vi "EPTxFPGA add-on test.vi"() -> ()   [LabVIEW 2019]
uses:
  <vilib>/Powertrain Controls/Device Drivers/Engine Position Tracking/EPTx/RevA/FPGA/Controls/EPTxSupervisor.ctl
  <vilib>/Powertrain Controls/Device Drivers/Engine Position Tracking/EPTx/RevA/FPGA/Controls/EPTxTooth.ctl
  <vilib>/Powertrain Controls/Device Drivers/Engine Position Tracking/EPTx/RevA/FPGA/Controls/EPTxConfig.ctl
  <vilib>/Platform/TimedLoop/XDataNode/timing_clust.ctl
  <vilib>/Platform/TimedLoop/XDataNode/nitl_modes.ctl
  <vilib>/Platform/TimedLoop/XDataNode/wakeup.ctl
  <vilib>/Powertrain Controls/Device Drivers/Engine Position Tracking/EPTx/RevA/FPGA/Controls/EPTxAAPControl.ctl
  <vilib>/Powertrain Controls/Device Drivers/Engine Position Tracking/EPTx/RevA/FPGA/Controls/EPTxSignals.ctl
  <vilib>/Powertrain Controls/Device Drivers/Engine Position Tracking/EPTx/RevA/FPGA/Controls/EPTxControl.ctl
  <vilib>/rvi/Emulation/niFpgaGetClockAttributes.vi
  <vilib>/rvi/Emulation/niFpgaSctlEmulationGetInTimedLoop.vi
  <vilib>/rvi/Emulation/niFpgaEmulationReportErrorSimple.vi
  <vilib>/rvi/Emulation/niFpgaCriticalErrorInLSC.vi
  <vilib>/rvi/eio/common/nirviEmuTemplateMethod_errors.vi
  <vilib>/rvi/interface/RandomDataEmulation/niFpgaRandomDataHandleErrors.vi
  <vilib>/eio/EIONode/EIONode.xnode
  <vilib>/rvi/DataTransferAndStorage/Container/XNode/niFpgaContainer.xnode
  <vilib>/rvi/interface/RandomDataEmulation/nirviRandomDataFpgaReadWriteTemplate.vi
  <vilib>/Platform/TimedLoop/XDataNode/XDataNode.xnode
  <vilib>/Powertrain Controls/Device Drivers/Engine Position Tracking/EPTx/RevA/FPGA/EPTx - RevA - FPGA.lvlib
  <vilib>/Platform/TimedLoop/XDataNode/XDNodeRunTimeDep.lvlib
panel:
  out "AvgSpeed":fxp<+/-,64,32>
  out "CADRate":fxp<+/-,64,32>
  out "HistoryCAD":fxp<+/-,64,32>
  out "MaxCAD":fxp<+/-,64,32>
  out "CurrentCAD":fxp<+/-,64,32>
  in  "Cylinder1_H_F [CAD]":fxp<+/-,64,32>
  in  "Cylinder1_H_R [CAD]":fxp<+/-,64,32>
  in  "Sim Rate":fxp<+/-,64,32>
  in  "EPTxConfig":T1
  out "EPTxTooth":T2
  out "EPTxSupervisor":T3
  in  "Enable":bool
  in  "FallingCAD":fxp<+/-,64,32>
  in  "Cylinder1_L_R [CAD]":fxp<+,18,11> format="%.11g"
  in  "Cylinder1_L_F [CAD]":fxp<+,18,11> format="%.11g"
  out "Sync":bool
  out "Config":bool
  out "Rcvg Primary":bool
  out "Stall":bool
  out "Overflow":bool
  out "Ratio Error":bool
  out "Pattern Error":bool
  out "Aux Warning":bool
  out "Watchdog Error":bool
  in  "Sync Enable":bool
  in  "Clear Errors":bool
  in  "Sim Enable":bool
  in  "Watchdog":bool
  in  "RisingCAD":fxp<+/-,64,32>
  in  "Eng_CurSpeed":fxp<+/-,64,32>
  in  "FXP27.5":fxp<+/-,27,5>
  out "FXP27.5 out":fxp<+/-,27,5>
  in  "FXP20.5":fxp<+/-,20,5>
  out "FXP20.5 out":fxp<+/-,20,5>
  in  "FXP16.7":fxp<+/-,16,7>
  out "FXP16.7 out":fxp<+/-,16,7>
  out "FXP64.32 out":fxp<+/-,64,32>
  out "FXP32.8 out":fxp<+/-,32,8>
  out "FXP16.5 out":fxp<+/-,16,5>
  out "FXP24.5 out":fxp<+/-,24,5>
  in  "FXP64.32":fxp<+/-,64,32>
  in  "FXP32.8":fxp<+/-,32,8>
  in  "FXP16.5":fxp<+/-,16,5>
  in  "FXP24.5":fxp<+/-,24,5>
  out "Boolean 2":bool=TRUE
  out "Fast timeout":bool
  out "Med timeout":bool
  out "Slow timeout":bool
  in  "I16":i16
  in  "I8":i8
  in  "I64":i64
  in  "I32":i32
  in  "U16":u16
  in  "U8":u8
  in  "U64":u64
  in  "U32":u32
  in  "SGL":sgl
  in  "Boolean":bool
  out "I16 out":i16
  out "I8 out":i8
  out "I64 out":i64
  out "I32 out":i32
  out "U16 out":u16
  out "U8 out":u8
  out "U64 out":u64
  out "U32 out":u32
  out "SGL out":sgl
  out "Boolean out":bool
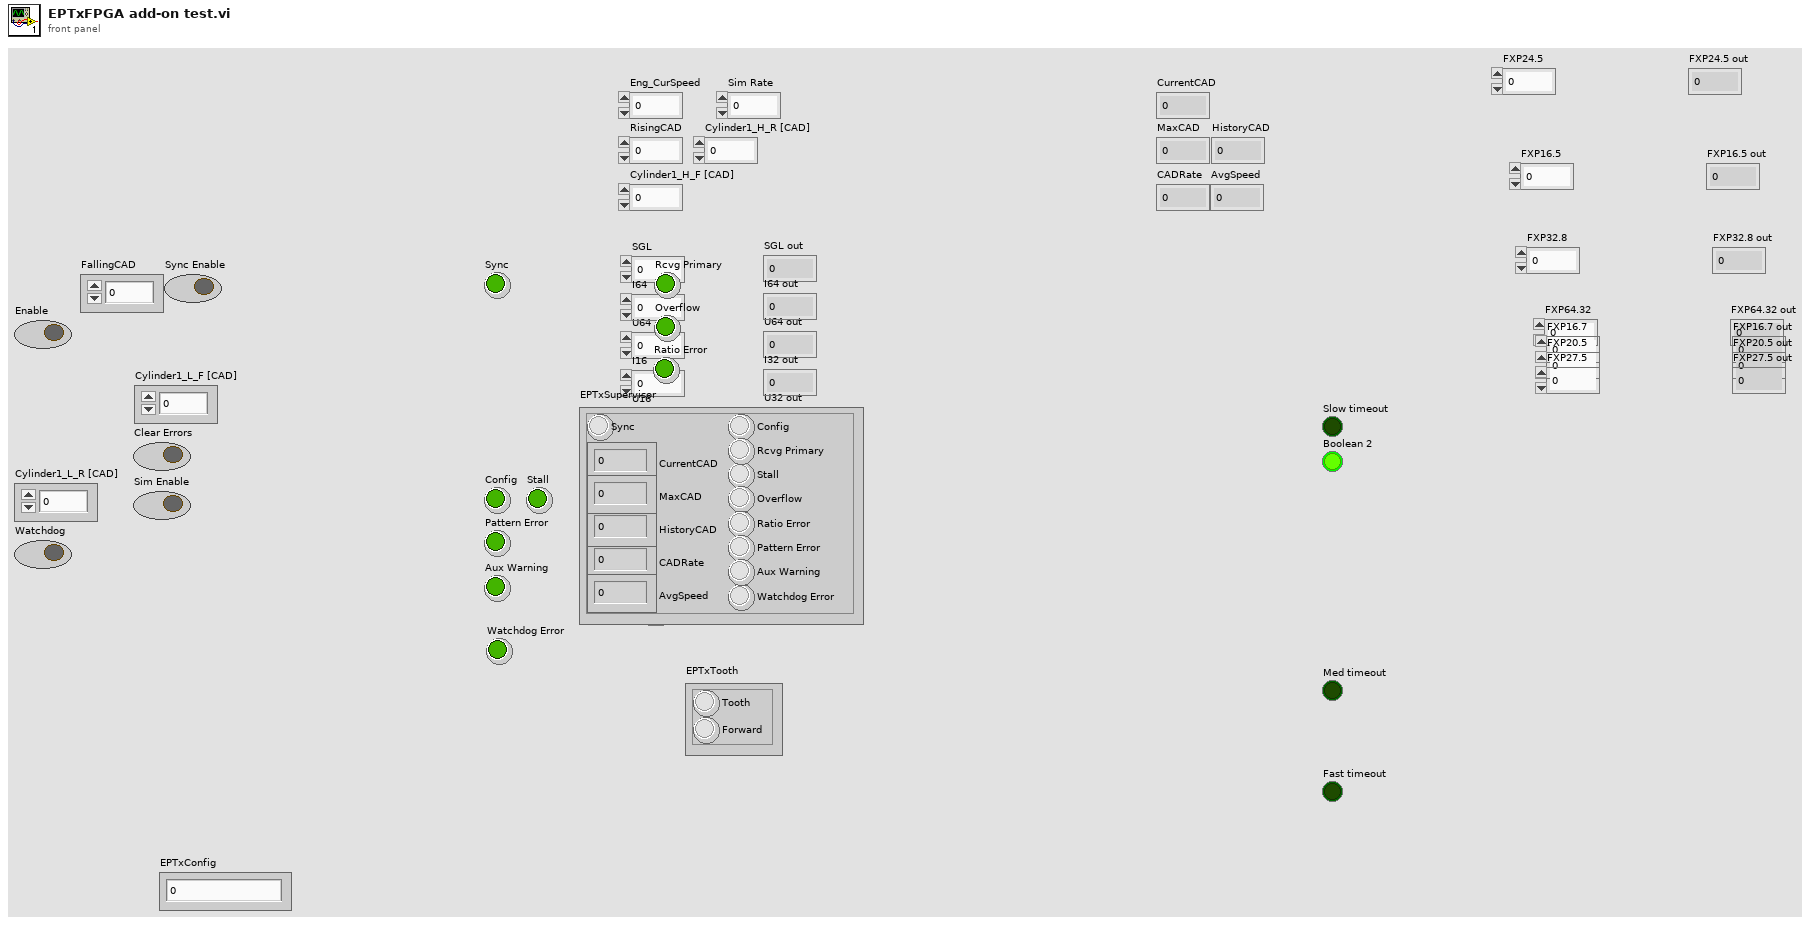
[diagram p1: front panel]
types:
  T1 = typedef "EPTx - RevA - FPGA.lvlib/EPTxConfig.ctl" = u64
  T2 = typedef "EPTx - RevA - FPGA.lvlib/EPTxTooth.ctl" = cluster{"Tooth":bool, "Forward":bool}
  T3 = typedef "EPTx - RevA - FPGA.lvlib/EPTxSupervisor.ctl" = cluster{"Sync":bool, "CurrentCAD":fxp<+,18,11>, "MaxCAD":fxp<+,11,11>, "HistoryCAD":fxp<+,11,11>, "CADRate":fxp<+,22,8>, "AvgSpeed":fxp<+,17,15>, "Config":bool, "Rcvg Primary":bool, "Stall":bool, "Overflow":bool, "Ratio Error":bool, "Pattern Error":bool, "Aux Warning":bool, "Watchdog Error":bool}
  T4 = typedef "EPTx - RevA - FPGA.lvlib/EPTxControl.ctl" = cluster{"Sync Enable":bool, "Clear Errors":bool, "Sim Enable":bool, "Sim Rate":fxp<+,24,6>, "Watchdog":bool}
  T5 = cluster{"Cylinder1_H_R [CAD]":fxp<+,18,11>, "Cylinder1_H_F [CAD]":fxp<+,18,11>, "Cylinder1_L_R [CAD]":fxp<+,18,11>, "Cylinder1_L_F [CAD]":fxp<+,18,11>}
  T6 = typedef "EPTx - RevA - FPGA.lvlib/EPTxAAPControl.ctl" = cluster{"Enable":bool, "RisingCAD":fxp<+,18,11>, "FallingCAD":fxp<+,18,11>}
  T7 = typedef "EPTx - RevA - FPGA.lvlib/EPTxSignals.ctl" = cluster{"Primary":bool, "Aux 1":bool, "Aux 2":bool, "Aux 3":bool, "Aux 4":bool}
  T8 = typedef "XDNodeRunTimeDep.lvlib/timing_clust.ctl" = cluster{"Expected End [f-1]":u64, "Actual End [f-1]":u64, "Finished Late? [f-1]":bool, "Expected End [i-1]":u64, "Actual End [i-1]":u64, "Finished Late? [i-1]":bool, "Expected Start [i]":u64, "Actual Start [i]":u64, "Expected Start [f]":u64, "Actual Start [f]":u64, "Source Name":string, "Structure Name":string, "Period":i64, "Deadline":i64, "Offset":i64, "Start":i64, "Priority":i32, "Timeout":i32, "Mode":T9, "Wakeup Reason":T10, "Error":errorcluster, "Source Type":string, "Secondary Source Type":string, "Global End Time":u64, "Global Start Time":u64, "Frame Duration":u64, "Iteration Duration":u64, "Assigned CPU":i32, "I/O Scan Engine Mode":u32}
  T9 = typedef "XDNodeRunTimeDep.lvlib/nitl_modes.ctl" = enum32{"No Change", "Process missed periods, maintain original phase", "Discard missed periods, maintain original phase", "Process missed periods, ignore original phase", "Discard missed periods, ignore original phase"}
  T10 = typedef "XDNodeRunTimeDep.lvlib/wakeup.ctl" = enum32{"Normal", "Aborted", "Asynchronous wakeup", "Timing source error", "Timed loop error", "Timeout"}
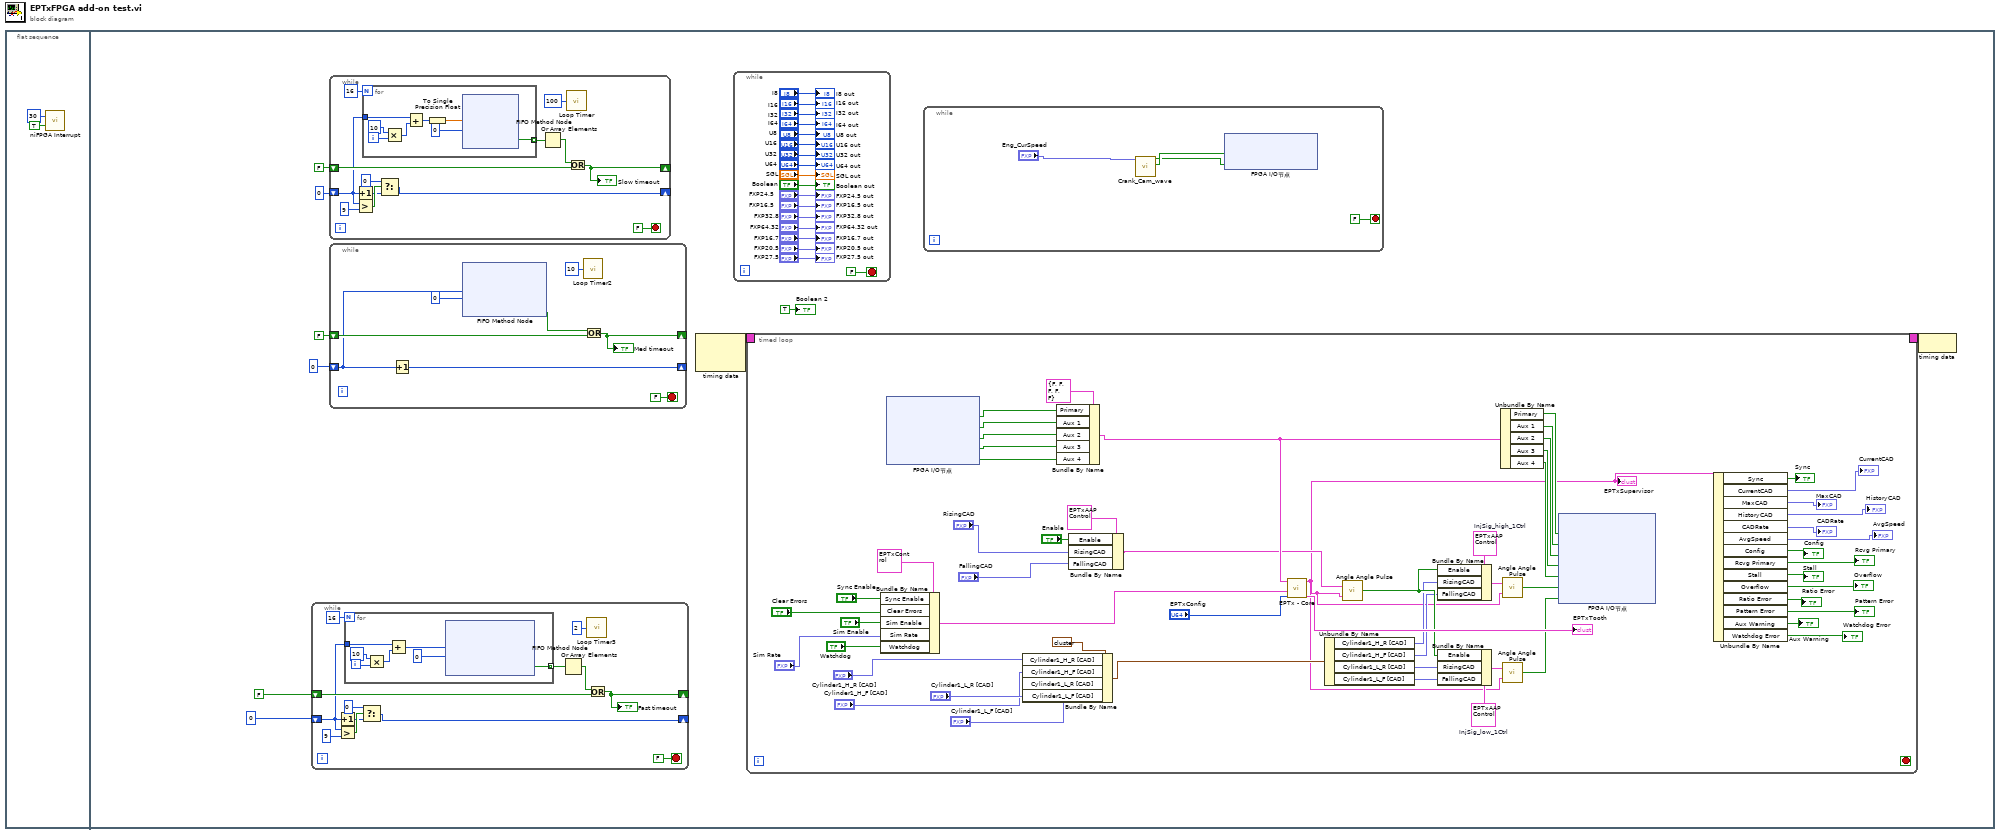
[diagram p0: block diagram]
diagram:
  n1 = flat-sequence {
    frame #0 {
      n2 = call <vilib>:"niFPGA Interrupt.vi"("Wait Until Cleared (F)"=TRUE, "IRQ Number (0)"=u8 30) -> ()  [unwired: 1 in]
    }
    frame #1 {
      n3 = while {
        shift-right: [w85] -> _
        shift-left: 0 ("t") -> [w78]
        shift-right: [w79] -> _
        shift-left: FALSE -> [w80]
        stop <- FALSE stop-if-true
        n4 = Increment(x=w78) -> (x+1=w83:i32)
        n5 = Greater?(x=w78, y=9) -> (0:w89:bool)
        n6 = for {
          N: 16 -> [_]
          tunnel: w78 -> [w97]
          tunnel: [w92] -> w82 mode=indexing
          i -> [w96]
          n7 = Multiply(x=10, y=w96) -> (x*y=w94:i32)
          n8 = Add(x=w97, y=w94) -> (x+y=w91:i32)
          n9 = xnode ("FIFO Method Node")("元素"=w91, "超时"=0 ("Timeout")) -> ("超时？"=w92:bool)  [unwired: 1 in, 1 out]
        }
        n10 = Select(t=0, s=w89, f=w83) -> (s? t:f=w85:i32)
        n11 = Or Array Elements ("数组元素或操作")(Boolean array=w82) -> (logical OR=w81:bool)
        n12 = call "Loop Timer3"("Count(uSec)"=u32 2) -> ()  [unwired: 1 out]
        n13 = Or(x=w81, y=w80) -> (x .or. y?=w79:bool)
        "Fast timeout" <- w79
      }
      n14 = while {
        shift-right: [w113] -> _
        shift-left: 0 ("t") -> [w106]
        shift-right: [w107] -> _
        shift-left: FALSE -> [w108]
        stop <- FALSE stop-if-true
        n15 = Increment(x=w106) -> (x+1=w111:i32)
        n16 = Greater?(x=w106, y=9) -> (0:w117:bool)
        n17 = for {
          N: 16 -> [_]
          tunnel: w106 -> [w126]
          tunnel: [w119] -> w110 mode=indexing
          i -> [w125]
          n18 = Multiply(x=10, y=w125) -> (x*y=w123:i32)
          n19 = Add(x=w126, y=w123) -> (x+y=w122:i32)
          n20 = To Single Precision Float(number=w122) -> (single precision float=w121:sgl)
          n21 = xnode ("FIFO Method Node")("元素"=w121, "超时"=0 ("Timeout")) -> ("超时？"=w119:bool)  [unwired: 1 in, 1 out]
        }
        n22 = Select(t=0, s=w117, f=w111) -> (s? t:f=w113:i32)
        n23 = Or Array Elements(Boolean array=w110) -> (logical OR=w109:bool)
        n24 = call "Loop Timer"("Count(uSec)"=u32 100) -> ()  [unwired: 1 out]
        n25 = Or(x=w109, y=w108) -> (x .or. y?=w107:bool)
        "Slow timeout" <- w107
      }
      n26 = while {
        shift-right: [w102] -> _
        shift-left: FALSE -> [w103]
        shift-right: [w98] -> _
        shift-left: u64 0 -> [w99]
        stop <- FALSE stop-if-true
        n27 = Increment(x=w99) -> (x+1=w98:u64)
        n28 = xnode ("FIFO Method Node")("元素"=w99, "超时"=0 ("Timeout")) -> ("超时？"=w100:bool)  [unwired: 1 in, 1 out]
        n29 = call "Loop Timer2"("Count(uSec)"=u32 10) -> ()  [unwired: 1 out]
        n30 = Or(x=w100, y=w103) -> (x .or. y?=w102:bool)
        "Med timeout" <- w102
      }
      n31 = node-c288() -> (w4:T8)  [unwired: 2 in]
      n32 = while {
        stop <- FALSE stop-if-true
        "I16 out" <- "I16"
        "I8 out" <- "I8"
        "I64 out" <- "I64"
        "I32 out" <- "I32"
        "U16 out" <- "U16"
        "U8 out" <- "U8"
        "U64 out" <- "U64"
        "U32 out" <- "U32"
        "SGL out" <- "SGL"
        "Boolean out" <- "Boolean"
        "FXP24.5 out" <- "FXP24.5"
        "FXP16.5 out" <- "FXP16.5"
        "FXP32.8 out" <- "FXP32.8"
        "FXP64.32 out" <- "FXP64.32"
        "FXP16.7 out" <- "FXP16.7"
        "FXP20.5 out" <- "FXP20.5"
        "FXP27.5 out" <- "FXP27.5"
      }
      n33 = timed-loop {
        timing: w4 -> [_]
        timing-out: [_] -> w3
        stop <- _ stop-if-true
        w60 = T6 {"Enable"=FALSE, "RisingCAD"=0.0, "FallingCAD"=0.0}  # InjSig_low_1Ctrl
        w61 = T6 {"Enable"=FALSE, "RisingCAD"=0.0, "FallingCAD"=0.0}  # InjSig_high_1Ctrl
        n34 = Bundle By Name(cluster=T4 {"Sync Enable"=FALSE, "Clear Errors"=FALSE, "Sim Enable"=FALSE, "Sim Rate"=0.0, "Watchdog"=FALSE} ("EPTxControl"), "Sync Enable"="Sync Enable", "Clear Errors"="Clear Errors", "Sim Enable"="Sim Enable", "Sim Rate"="Sim Rate", "Watchdog"="Watchdog") -> (w21:T4)
        n35 = xnode "FPGA I/O节点"() -> ("Connector1/DIO0"=w49:bool, "Connector1/DIO1"=w48:bool, "Connector1/DIO2"=w47:bool, "Connector1/DIO3"=w46:bool, "Connector1/DIO4"=w45:bool)  [unwired: 5 in, 5 out]
        n36 = Bundle By Name(cluster=T5 {"Cylinder1_H_R [CAD]"=0.0, "Cylinder1_H_F [CAD]"=0.0, "Cylinder1_L_R [CAD]"=0.0, "Cylinder1_L_F [CAD]"=0.0} ("CylinderSig_1"), "Cylinder1_H_R [CAD]"="Cylinder1_H_R [CAD]", "Cylinder1_H_F [CAD]"="Cylinder1_H_F [CAD]", "Cylinder1_L_R [CAD]"="Cylinder1_L_R [CAD]", "Cylinder1_L_F [CAD]"="Cylinder1_L_F [CAD]") -> (w37:T5)
        n37 = Bundle By Name(cluster=T7 {"Primary"=FALSE, "Aux 1"=FALSE, "Aux 2"=FALSE, "Aux 3"=FALSE, "Aux 4"=FALSE} ("EPTxSignals"), "Primary"=w49, "Aux 1"=w48, "Aux 2"=w47, "Aux 3"=w46, "Aux 4"=w45) -> (w50:T7)
        n38 = Bundle By Name(cluster=T6 {"Enable"=FALSE, "RisingCAD"=0.0, "FallingCAD"=0.0} ("AAPControl_1str"), "Enable"="Enable", "RisingCAD"="RisingCAD", "FallingCAD"="FallingCAD") -> (w41:T6)
        n39 = call <vilib>:"EPTx - Core.vi"("EPTxConfig"="EPTxConfig", "EPTxControl"=w21, "EPTxSignals"=w50) -> ("EPTxTooth"=→"EPTxTooth":T2, "EPTxSupervisor"=w36:T3)  [unwired: 7 in]
        "EPTxSupervisor" <- w36
        n40 = Unbundle By Name(w37) -> ("Cylinder1_H_R [CAD]"=w57:fxp<+,18,11>, "Cylinder1_H_F [CAD]"=w56:fxp<+,18,11>, "Cylinder1_L_R [CAD]"=w55:fxp<+,18,11>, "Cylinder1_L_F [CAD]"=w54:fxp<+,18,11>)
        n41 = call <vilib>:"Angle Angle Pulse.vi"("EPTxSupervisor"=w36, "AAPControl"=w41) -> ("AAP"=w58:bool)
        n42 = Bundle By Name(cluster=w61, "Enable"=w58, "RisingCAD"=w57, "FallingCAD"=w56) -> (w62:T6)
        n43 = Bundle By Name(cluster=w60, "Enable"=w58, "RisingCAD"=w55, "FallingCAD"=w54) -> (w59:T6)
        n44 = Unbundle By Name(w50) -> ("Primary"=w67:bool, "Aux 1"=w66:bool, "Aux 2"=w65:bool, "Aux 3"=w64:bool, "Aux 4"=w63:bool)
        n45 = call <vilib>:"Angle Angle Pulse.vi"("EPTxSupervisor"=w36, "AAPControl"=w62) -> ("AAP"=w53:bool)
        n46 = call <vilib>:"Angle Angle Pulse.vi"("EPTxSupervisor"=w36, "AAPControl"=w59) -> ("AAP"=w52:bool)
        n47 = xnode "FPGA I/O节点"("Connector0/DIO4"=w67, "Connector0/DIO5"=w66, "Connector0/DIO6"=w65, "Connector0/DIO7"=w64, "Connector0/DIO8"=w63, "Connector0/DIO9"=w53, "Connector0/DIO10"=w52) -> ()  [unwired: 7 in, 7 out]
        n48 = Unbundle By Name(w36) -> ("Sync"=→"Sync":bool, "CurrentCAD"=→"CurrentCAD":fxp<+,18,11>, "MaxCAD"=→"MaxCAD":fxp<+,11,11>, "HistoryCAD"=→"HistoryCAD":fxp<+,11,11>, "CADRate"=→"CADRate":fxp<+,22,8>, "AvgSpeed"=→"AvgSpeed":fxp<+,17,15>, "Config"=→"Config":bool, "Rcvg Primary"=→"Rcvg Primary":bool, "Stall"=→"Stall":bool, "Overflow"=→"Overflow":bool, "Ratio Error"=→"Ratio Error":bool, "Pattern Error"=→"Pattern Error":bool, "Aux Warning"=→"Aux Warning":bool, "Watchdog Error"=→"Watchdog Error":bool)
      }
      n49 = while {
        stop <- FALSE stop-if-true
        n50 = call "Crank_Cam_wave.vi"("当前转速"="Eng_CurSpeed") -> ("曲轴"=w76:bool, "凸轮轴"=w75:bool)  [unwired: 9 in]
        n51 = xnode "FPGA I/O节点"("Connector0/DIO0"=w76, "Connector0/DIO1"=w75) -> ()  [unwired: 2 in, 2 out]
      }
      n52 = node-c288(w3) -> ()
      "Boolean 2" <- TRUE
    }
  }
